vi "thread queue fglbl_AuditHMI.vi"(8 "error in (no error)":errorcluster, 10 "Station AuditHMI Thread ID":T1, 11 "action":T2) -> (0 "error out":errorcluster, 2 "all queues":refnum<queue>[](array[refnum]), 3 "queue out":refnum<queue>)   [LabVIEW 2012]
uses:
  typedefs/interthread message.ctl
  typedefs/state queue fglbl actions.ctl
  typedefs/station AuditHMI thread IDs.ctl
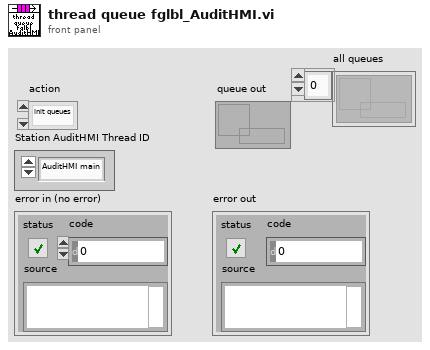
[diagram p1: front panel]
types:
  T1 = typedef "station AuditHMI thread IDs.ctl" = enum16{"AuditHMI main", "tcp comms"}
  T2 = typedef "state queue fglbl actions.ctl" = enum16{"init queues", "get queue ref", "destroy queues"}
  T3 = typedef "interthread message.ctl" = cluster{"destination state":string, "data":variant}
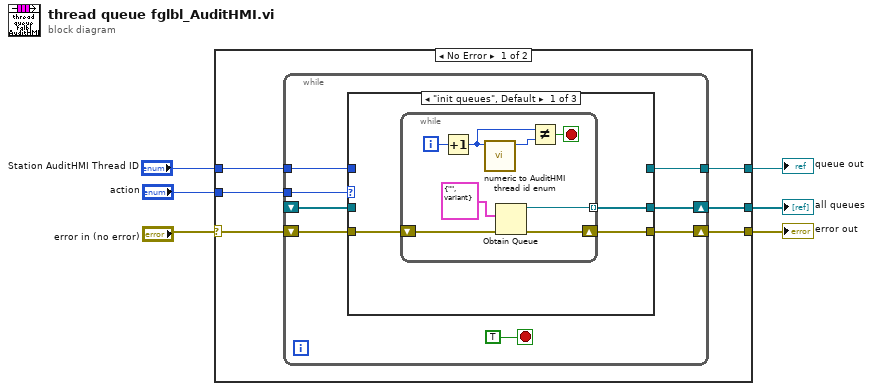
[diagram p0: block diagram]
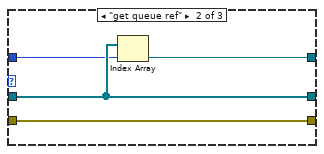
[diagram p2: hidden frame]
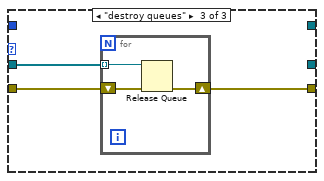
[diagram p3: hidden frame]
diagram:
  n1 = case shown="No Error" "error in (no error)" {
    selector: "error in (no error)" -> [w12 w42]
    tunnel: [w11 w42] -> w4
    tunnel: "action" -> [w10 _]
    tunnel: "Station AuditHMI Thread ID" -> [w9 _]
    tunnel: [w8 _] -> w6
    tunnel: [w7 _] -> w2
    frame No Error {
      n2 = while {
        shift-right: [w17] -> w11
        shift-left: w12 -> [w18]
        tunnel: w10 -> [w19]
        tunnel: w9 -> [w14]
        shift-right: [w16] -> w7
        shift-left: _ -> [w15]
        tunnel: [w13] -> w8
        stop <- TRUE stop-if-true
        n3 = case shown="\"init queues\", Default" w19 {
          tunnel: w18 -> [w23 w32 w37]
          tunnel: [w22 w32 w36] -> w17
          tunnel: [w21 w35 _] -> w16
          tunnel: w15 -> [_ w35 w38]
          tunnel: w14 -> [_ w34 _]
          tunnel: [_ w33 _] -> w13
          frame "init queues", Default {
            n4 = while {
              shift-right: [w29] -> w22
              shift-left: w23 -> [w30]
              tunnel: [w28] -> w21 mode=indexing
              i -> [w26]
              stop <- w24 stop-if-true
              n5 = Increment(x=w26) -> (x+1=w25:i32)
              n6 = call "numeric to AuditHMI thread id enum.vi"("Numeric"=w25) -> ("Station cDAQ Thread Queues out"=w27:T1)  [unwired: 10 in]
              n7 = Obtain Queue(element data type=T3 {"destination state"="", "data"=variant}, error in (no error)=w30) -> (queue out=w28:refnum<queue>, error out=w29:errorcluster)  [unwired: 3 in, 1 out]
              n8 = Not Equal?(x=w25, y=w27) -> (x != y?=w24:bool)
            }
          }
          frame "get queue ref" {
            n9 = Index Array(array=w35, index=w34) -> (element=w33:refnum<queue>)
          }
          frame "destroy queues" {
            n10 = for {
              tunnel: w38 -> [w41] mode=indexing
              shift-right: [w39] -> w36
              shift-left: w37 -> [w40]
              n11 = Release Queue(queue=w41, error in (no error)=w40) -> (error out=w39:errorcluster)  [unwired: 1 in, 2 out]
            }
          }
        }
      }
    }
    frame Error {
    }
  }
  "queue out" <- w6
  "error out" <- w4
  "all queues" <- w2
